vi "GetAttachedTaikoSerials.vi"(8 "error in (no error)":errorcluster) -> (2 "Array 2":i32[](array[numeric]), 3 "Array":string[](array[string]))   [LabVIEW 2019]
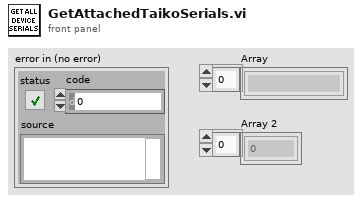
[diagram p1: front panel]
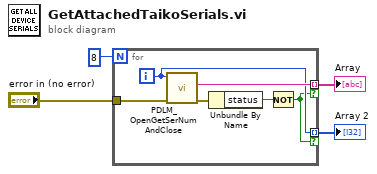
[diagram p0: block diagram]
diagram:
  n1 = for {
    N: 8 -> [_]
    tunnel: [w10] -> w4 mode=indexing if=w6
    tunnel: "error in (no error)" -> [w9]
    tunnel: [w8] -> w3 mode=indexing if=w6
    i -> [w8]
    n2 = call <userlib>:"PDLM_OpenGetSerNumAndClose.vi"("error in (no error)"=w9, "USBIdx"=w8) -> ("error out"=w5:errorcluster, "SerNo"=w10:string)  [unwired: 7 in, 1 out]
    n3 = Unbundle By Name(w5) -> ("status"=w7:bool)
    n4 = Not(x=w7) -> (.not. x?=w6:bool)
  }
  "Array" <- w4
  "Array 2" <- w3
